vi "util.environment.vi"(8 "error in":errorcluster, 9 "Operation (Get)":enum16{"get", "set"}(ring), 11 "ENV in":T1) -> (0 "error out":errorcluster, 3 "ENV out":T1)   [LabVIEW 2024]
uses:
  controls/typeEnv.ctl
  controls/ini-key.ctl
  controls/typePathSelector.ctl
  <vilib>/Utility/error.llb/Clear Errors.vi
  <vilib>/Utility/libraryn.llb/Create Directory Recursive.vi
  <vilib>/Utility/config.llb/Write Key (String).vi
  <vilib>/Utility/config.llb/NI_LVConfig.lvlib
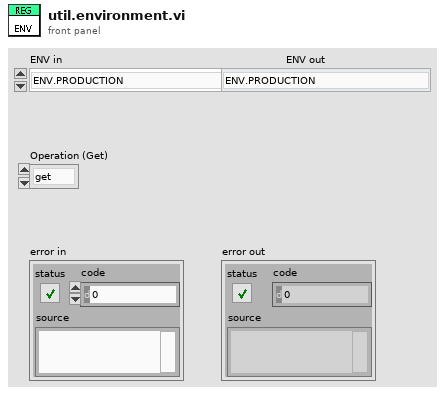
[diagram p1: front panel]
types:
  T1 = typedef "typeEnv.ctl" = enum16{"ENV.PRODUCTION", "ENV.TEST.NO-HW", "ENV.TEST.SINGLE-01", "ENV.TEST.SINGLE-02", "ENV.TEST.SINGLE-02 AI 0", "ENV.TEST.SINGLE-03"}
  T2 = typedef "typePathSelector.ctl" = enum16{"DIR_PROCS", "DIR_CONFIG", "DIR_TEMPLATE", "DIR_IO_FILE", "DIR_RECORD", "DIR_LOG", "DIR_RUNTIME", "DIR_PRESET", "DIR_INI"}
  T3 = typedef "ini-key.ctl" = enum16{"INI.PROJECT_NAME", "INI.ENV", "INI.ENG.SERIAL", "INI.ENG.INTERVAL_MS", "INI.LOCAL.LONGITUDE", "INI.LOCAL.LATITUDE", "INI.LOCAL.TIMEZONE"}
  T4 = typedef "NI_LVConfig.lvlib/Config Data RefNum.ctl" = refnum<k1>
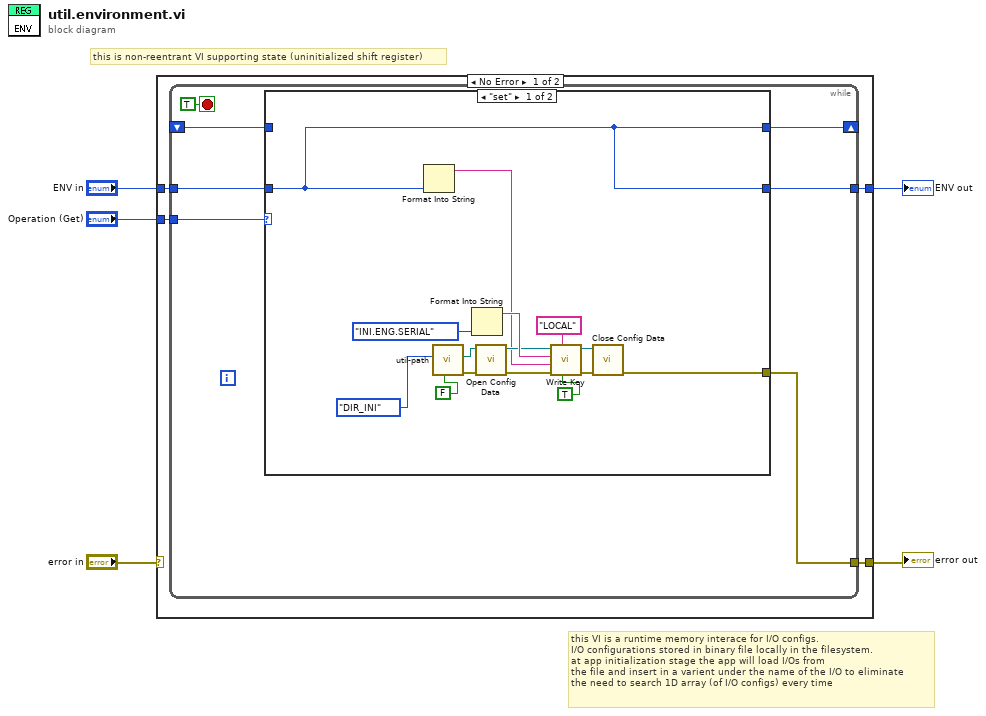
[diagram p0: block diagram]
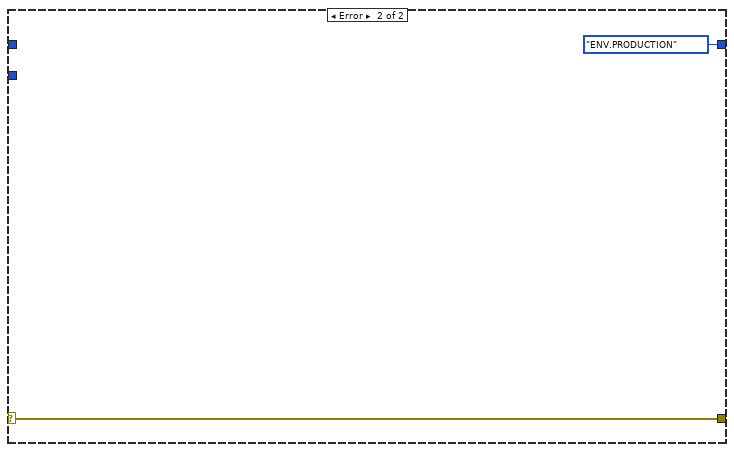
[diagram p3: hidden frame]
diagram:
  # "this is non-reentrant VI supporting state (uninitialized shift register)"
  # "this VI is a runtime memory interace for I/O configs. \nI/O configurations stored in binary file locally in the filesystem.\nat app initialization stage the app will load I/Os from\nthe file and insert in a varient under the name of the I/O to eliminate \nthe need to search 1D array (of I/O configs) every time"
  n1 = case shown="No Error" "error in" {
    selector: "error in" -> [_ w34]
    tunnel: "ENV in" -> [w9 _]
    tunnel: "Operation (Get)" -> [w8 _]
    tunnel: [w7 typeEnv."ENV.PRODUCTION" ("ENV in")] -> w3
    tunnel: [w6 w34] -> w2
    frame No Error {
      n2 = while {
        tunnel: w8 -> [w13]
        tunnel: w9 -> [w16]
        tunnel: [w12] -> w7
        shift-right: [w14] -> _
        shift-left: _ -> [w15]
        tunnel: [w10] -> w6
        stop <- TRUE stop-if-true
        n3 = case shown="\"set\"" w13 {
          tunnel: w16 -> [w17 _]
          tunnel: w15 -> [_ w32]
          tunnel: [w17 w32] -> w14
          tunnel: [w17 w32] -> w12
          tunnel: [w18 _] -> w10
          frame "set" {
            n4 = Format Into String(w17) -> (resulting string=w19:string)  [unwired: 3 in, 1 out]
            n5 = call "util-path.vi"("Create Folders?(F)"=FALSE, "Selected Folder (PROCS)"=typePathSelector."DIR_INI" ("Selected Folder (PROCEDURE_DIR)")) -> ("error out"=w30:errorcluster, "SelectedPath"=w28:path)  [unwired: 5 in, 3 out]
            n6 = Format Into String(ini-key."INI.ENG.SERIAL" ("keys")) -> (resulting string=w31:string)  [unwired: 3 in, 1 out]
            n7 = call <vilib>:"Open Config Data.vi"("error in (no error)"=w30, "configuration file path"=w28) -> ("error out"=w29:errorcluster, "refnum"=w27:T4)  [unwired: 7 in, 1 out]
            n8 = call-poly <vilib>:"Write Key.vi"("write raw string? (F)"=TRUE, "section"="LOCAL", "error in (no error)"=w29, "value"=w19, "key"=w31, "refnum"=w27) -> ("error out"=w26:errorcluster, "refnum out"=w25:T4)  [unwired: 3 in, 1 out]
            n9 = call <vilib>:"Close Config Data.vi"("error in (no error)"=w26, "refnum"=w25) -> ("error out"=w18:errorcluster)  [unwired: 8 in, 1 out]
          }
          frame "get", Default {
          }
        }
      }
    }
    frame Error {
    }
  }
  "error out" <- w2
  "ENV out" <- w3
